vi "array.vi"() -> ()   [LabVIEW 2020]
panel:
  out "initialized array":dbl[][](array[numeric])
  out "appended array":string[](array[string])
  out "transposed array":i32[][](array[numeric])
  out "array w/ subset deleted 2":i32[][](array[numeric])
  out "deleted portion":string[](array[string])
  out "array w/ subset deleted":string[](array[string])
  out "output array 2":string[](array[string])
  out "element":i32
  out "output array":i32[][](array[numeric])
  out "size(s) 2":i32
  out "size(s)":i32[](array[numeric])
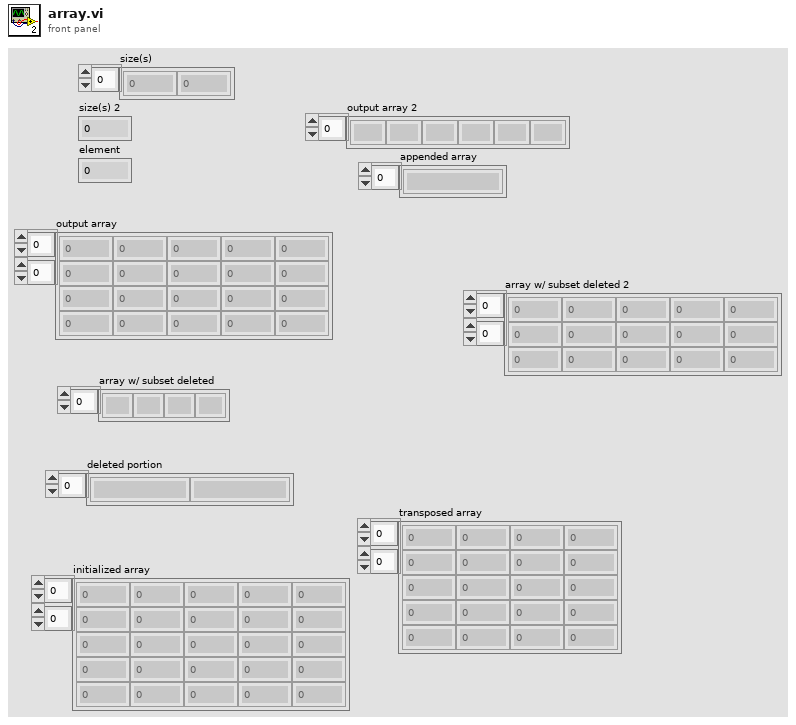
[diagram p1: front panel]
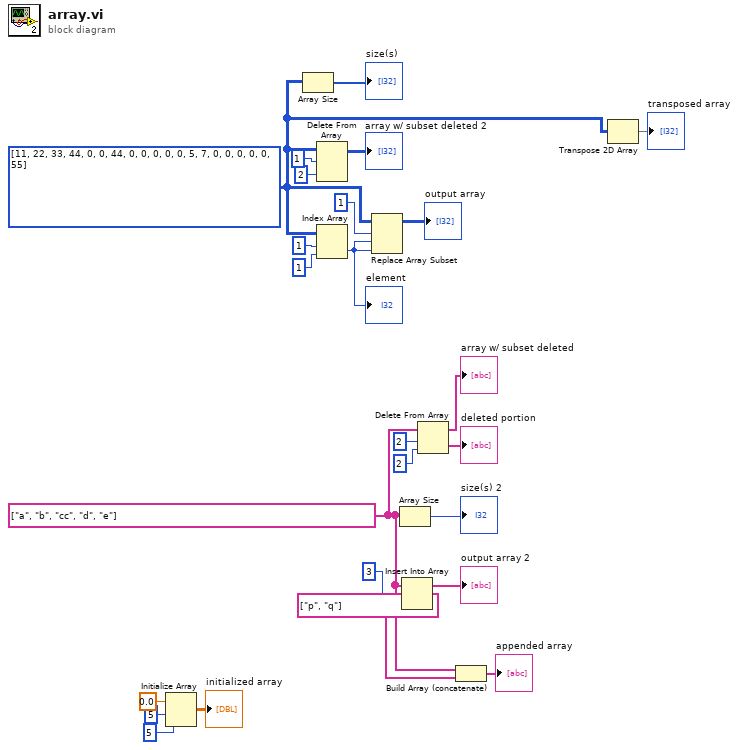
[diagram p0: block diagram]
diagram:
  w6 = string[] ["p", "q"]
  w9 = i32[][] [[11, 22, 33, 44, 0], [0, 44, 0, 0, 0], [0, 0, 5, 7, 0], [0, 0, 0, 0, 55]]
  w7 = string[] ["a", "b", "cc", "d", "e"]
  n1 = Initialize Array(0.0 ("element"), 5 ("dimension size"), 5 ("dimension size")) -> (→"initialized array":dbl[][])
  n2 = Array Size(array=w9) -> (size(s)=→"size(s)":i32[])
  n3 = Delete From Array(array=w9, length=1 ("index"), index (row)=2) -> (array with subset deleted=→"array w/ subset deleted 2":i32[][])  [unwired: 1 in, 1 out]
  n4 = Index Array(array=w9, index (row)=1, index (col)=1 ("disabled index (col)")) -> (element=w21:i32)
  "element" <- w21
  n5 = Replace Array Subset(array=w9, new element=w21, index (row)=1, index (col)=w21) -> (→"output array":i32[][])
  n6 = Array Size(array=w7) -> (size(s)=→"size(s) 2":i32)
  n7 = Insert Into Array(array=w7, index=3, new element=w6) -> (→"output array 2":string[])
  n8 = Delete From Array(array=w7, length=2, index=2) -> (deleted portion=→"deleted portion":string[], array with subset deleted=→"array w/ subset deleted":string[])
  n9 = Build Array (concatenate)(w7, w6) -> (→"appended array":string[])
  n10 = Transpose 2D Array(2D array=w9) -> (transposed array=→"transposed array":i32[][])
